vi "Poll Storage Line Valve Control.vi"(8 "error in (no error)":errorcluster, 11 "Storage Line in":refnum<class "Storage Line.lvclass">) -> ()   [LabVIEW 2015, in "cRIO-Carbondioxide.lvlib" / "CO2-Actor.lvlib" / "Storage Line.lvclass"]
uses:
  Storage Line.lvclass
  Storage Line.lvclass/Storage Line.ctl
  <vilib>/ActorFramework/Actor/Actor.lvclass/Actor.ctl
  <vilib>/ActorFramework/Message Enqueuer/Message Enqueuer.lvclass/Message Enqueuer.ctl
  Storage Line Messages/Handle Line Control Change Msg/Handle Line Control Change Msg.lvclass/Handle Line Control Change Msg.ctl
  <vilib>/ActorFramework/Actor/Read Self Enqueuer.vi
  <vilib>/ActorFramework/Message Enqueuer/Enqueue.vi
  <vilib>/ActorFramework/Message Enqueuer/Init from Existing Queue.vi
  <vilib>/ActorFramework/Message Priority Queue/Priority Enqueue.vi
  <vilib>/ActorFramework/Actor/Actor.lvclass
  <vilib>/ActorFramework/Message Enqueuer/Message Enqueuer.lvclass
  Storage Line Messages/Handle Line Control Change Msg/Handle Line Control Change Msg.lvclass
  CO2 Actor/CO2 Actor.lvclass
  cRIO-CO2/cRIO-CO2.lvclass
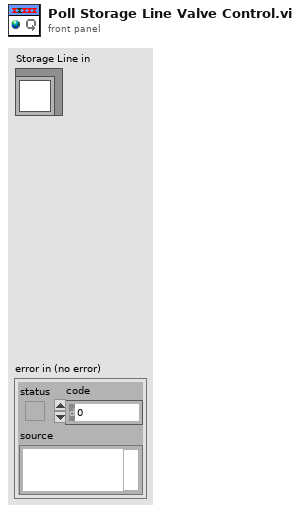
[diagram p1: front panel]
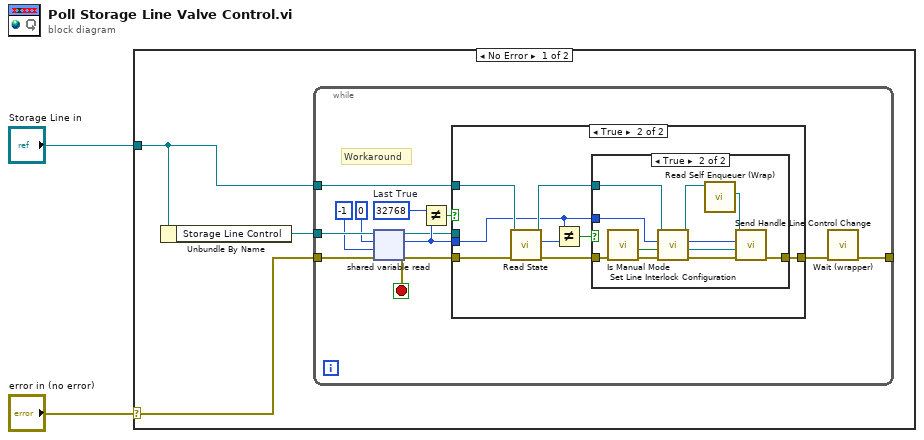
[diagram p0: block diagram]
diagram:
  n1 = case shown="No Error" "error in (no error)" {
    selector: "error in (no error)" -> [w4 _]
    tunnel: "Storage Line in" -> [w3 _]
    frame No Error {
      n2 = Unbundle By Name(w3) -> ("Storage Line Control"=w5:refnum<k21>)
      n3 = while {
        tunnel: w4 -> [w17]
        tunnel: w5 -> [w16]
        tunnel: w3 -> [w10]
        tunnel: [w6] -> _
        stop <- w8 stop-if-true
        w11 = u16 32768  # Last True
        # "Workaround"
        n4 = shared-variable-read(w16, w17, -1 ("timeout ms"), u16 0) -> (w9:refnum<k21>, w8:errorcluster, w12:u16)  [unwired: 2 out]
        n5 = Not Equal?(x=w11, y=w12) -> (x != y?=w13:bool)
        n6 = case shown="True" w13 {
          tunnel: [w18 w26] -> w7
          tunnel: w8 -> [w18 w25]
          tunnel: w12 -> [_ w21]
          tunnel: w10 -> [_ w23]
          tunnel: w9 -> [_ _]
          frame False {
            # "The value is\nfor refreshing\npurposes.\nIgnore"
          }
          frame True {
            n7 = call "Read State.vi"("error in (no error)"=w25, "Storage Line in"=w23) -> ("error out"=w24:errorcluster, "State"=w20:u16, "Storage Line out"=w22:refnum<class "Storage Line.lvclass">)  [unwired: 5 in, 2 out]
            n8 = Not Equal?(x=w21, y=w20) -> (x != y?=w19:bool)
            n9 = case shown="True" w19 {
              tunnel: [w27 w38] -> w26
              tunnel: w21 -> [_ w31]
              tunnel: w24 -> [w27 w29]
              tunnel: w22 -> [_ w28]
              frame False {
              }
              frame True {
                n10 = call "Is Manual Mode.vi"("error in (no error)"=w29) -> ("error out"=w37:errorcluster, "Manual Mode?"=w36:bool)  [unwired: 9 in]
                n11 = call "Set Line Interlock Configuration.vi"("error in (no error)"=w37, "Manual Mode (False)"=w36, "Bit Field In"=w31, "Storage Line in"=w28) -> ("error out"=w35:errorcluster, "Interlock Chain out"=w30:refnum<class "Interlock Chain.lvclass">, "Bit Field out"=w32:u16, "Storage Line out"=w33:refnum<class "Storage Line.lvclass">)  [unwired: 4 in]
                n12 = call "Read Self Enqueuer (Wrap).vi"("CO2 Actor in"=w33) -> ("Actor Framework:Message Enqueuer"=w34:refnum<class "Message Enqueuer.lvclass">)  [unwired: 9 in, 1 out]
                n13 = call "Send Handle Line Control Change.vi"("error in (no error)"=w35, "Interlock Chain"=w30, "Requested Bitfield"=w32, "Message Enqueuer"=w34) -> ("error out"=w38:errorcluster)  [unwired: 6 in, 1 out]
              }
            }
          }
        }
        n14 = call "Wait (wrapper).vi"("error in (no error)"=w7) -> ("error out"=w6:errorcluster)  [unwired: 10 in]
      }
    }
    frame Error {
    }
  }
